vi "FPGA_Set Digital Input.vi"(11 "Digital Input In":T1={"DI 0"="RMC/DIO15", "DI 1"="RMC/DIO47", "DI 2"="RMC/DIO46", "DI 3"="RMC/DIO79", "DI 4"="RMC/DIO63", "DI 5"="RMC/DIO14", "DI 6"="RMC/DIO78", "DI 7"="RMC/DIO31", "DI 8"="RMC/DIO95", "DI 9"="RMC/DIO13", "DI 10"="RMC/DIO45", "DI 11"="RMC/DIO30"}) -> (3 "Digital Input Out":T1={"DI 0"="RMC/DIO15", "DI 1"="RMC/DIO47", "DI 2"="RMC/DIO46", "DI 3"="RMC/DIO79", "DI 4"="RMC/DIO63", "DI 5"="RMC/DIO14", "DI 6"="RMC/DIO78", "DI 7"="RMC/DIO31", "DI 8"="RMC/DIO95", "DI 9"="RMC/DIO13", "DI 10"="RMC/DIO45", "DI 11"="RMC/DIO30"})   [LabVIEW 2018]
uses:
  Data Def/FPGA_Digital Input.ctl
  <vilib>/rvi/eio/common/nirviEmuTemplateMethod_errors.vi
  <vilib>/eio/EIOMethodNode/EIOMethodNode.xnode
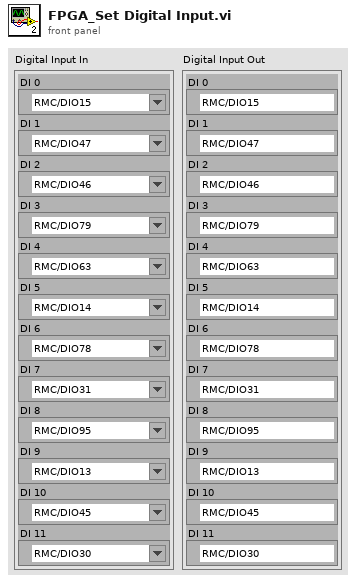
[diagram p1: front panel]
types:
  T1 = typedef "FPGA_Digital Input.ctl" = cluster{"DI 0":refnum<k21>, "DI 1":refnum<k21>, "DI 2":refnum<k21>, "DI 3":refnum<k21>, "DI 4":refnum<k21>, "DI 5":refnum<k21>, "DI 6":refnum<k21>, "DI 7":refnum<k21>, "DI 8":refnum<k21>, "DI 9":refnum<k21>, "DI 10":refnum<k21>, "DI 11":refnum<k21>}
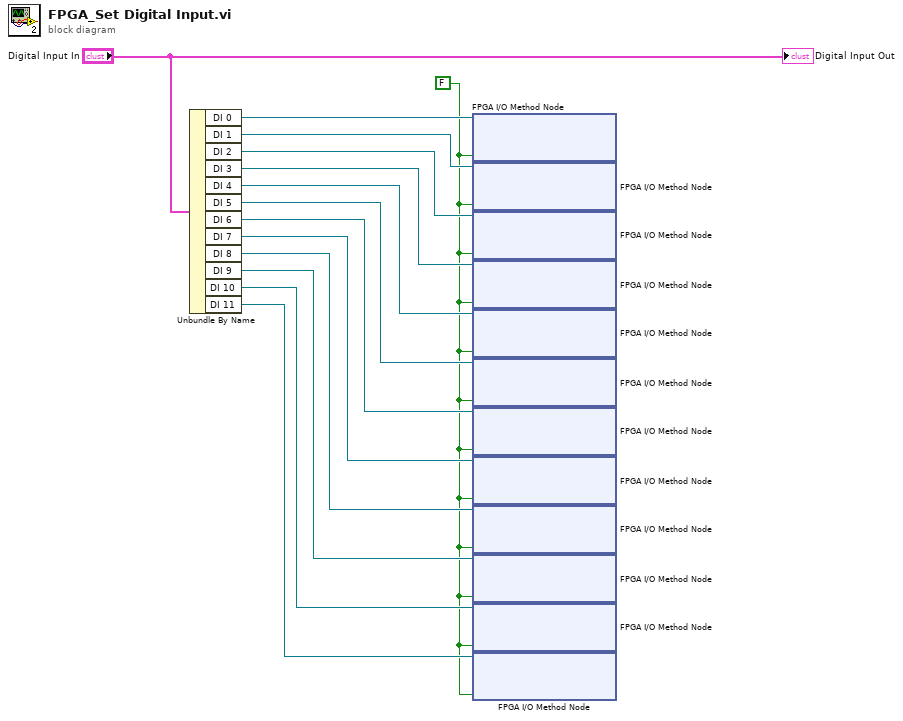
[diagram p0: block diagram]
diagram:
  w2 = FALSE ("Enable")
  n1 = Unbundle By Name("Digital Input In") -> ("DI 0"=w14:refnum<k21>, "DI 1"=w13:refnum<k21>, "DI 2"=w12:refnum<k21>, "DI 3"=w11:refnum<k21>, "DI 4"=w10:refnum<k21>, "DI 5"=w9:refnum<k21>, "DI 6"=w8:refnum<k21>, "DI 7"=w7:refnum<k21>, "DI 8"=w6:refnum<k21>, "DI 9"=w5:refnum<k21>, "DI 10"=w4:refnum<k21>, "DI 11"=w3:refnum<k21>)
  n2 = xnode "FPGA I/O Method Node"("FPGA I/O In"=w14, "Enable"=w2) -> ()  [unwired: 1 out]
  n3 = xnode "FPGA I/O Method Node"("FPGA I/O In"=w13, "Enable"=w2) -> ()  [unwired: 1 out]
  n4 = xnode "FPGA I/O Method Node"("FPGA I/O In"=w12, "Enable"=w2) -> ()  [unwired: 1 out]
  n5 = xnode "FPGA I/O Method Node"("FPGA I/O In"=w11, "Enable"=w2) -> ()  [unwired: 1 out]
  n6 = xnode "FPGA I/O Method Node"("FPGA I/O In"=w10, "Enable"=w2) -> ()  [unwired: 1 out]
  n7 = xnode "FPGA I/O Method Node"("FPGA I/O In"=w9, "Enable"=w2) -> ()  [unwired: 1 out]
  n8 = xnode "FPGA I/O Method Node"("FPGA I/O In"=w8, "Enable"=w2) -> ()  [unwired: 1 out]
  n9 = xnode "FPGA I/O Method Node"("FPGA I/O In"=w7, "Enable"=w2) -> ()  [unwired: 1 out]
  n10 = xnode "FPGA I/O Method Node"("FPGA I/O In"=w6, "Enable"=w2) -> ()  [unwired: 1 out]
  n11 = xnode "FPGA I/O Method Node"("FPGA I/O In"=w5, "Enable"=w2) -> ()  [unwired: 1 out]
  n12 = xnode "FPGA I/O Method Node"("FPGA I/O In"=w4, "Enable"=w2) -> ()  [unwired: 1 out]
  n13 = xnode "FPGA I/O Method Node"("FPGA I/O In"=w3, "Enable"=w2) -> ()  [unwired: 1 out]
  "Digital Input Out" <- "Digital Input In"
